vi "Configure Open Lead Detection.vi"(7 "Enable Open Lead Detection (F: Disable)":bool, 8 "error in (no error)":errorcluster, 9 "Channel List(\"\")":string, 10 "Function (5: 4-wire resistance)":i32(ring)=5 items=["4-wire Resistance"=5, "Temperature"=8], 11 "VISA resource name":refnum<visa-resource-name>) -> (0 "error out":errorcluster, 3 "VISA resource name out":refnum<visa-resource-name>)   [LabVIEW 2019, in "Keithley DMM6500 DAQ6500 Series.lvlib"]
doc: "Determines if the detection of open leads is enabled or disabled."
uses:
  Keithley DMM6500 DAQ6500 Series.lvlib
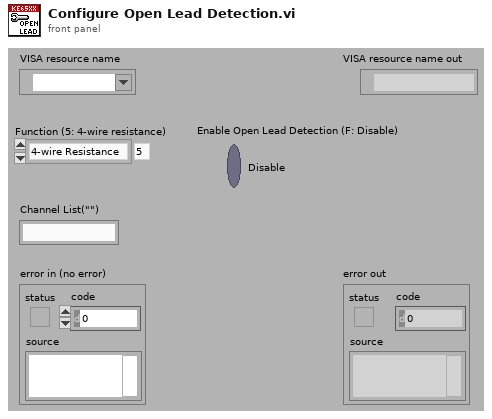
[diagram p1: front panel]
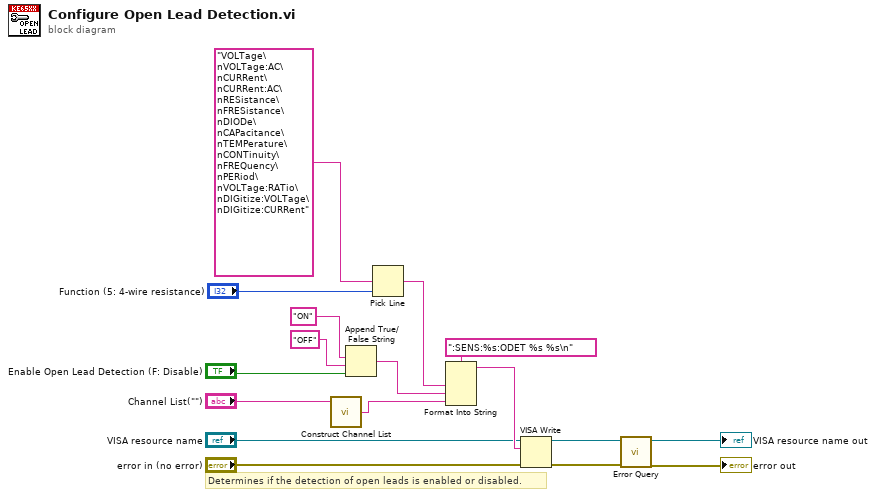
[diagram p0: block diagram]
diagram:
  # "Determines if the detection of open leads is enabled or disabled."
  n1 = call "Construct Channel List.vi"("Channel List"="Channel List(\"\")") -> ("Channel List String"=w4:string)  [unwired: 2 in]
  n2 = Append True/False String(1:"Enable Open Lead Detection (F: Disable)", 2:"OFF", 3:"ON") -> (0:w13:string)  [unwired: 1 in]
  n3 = Pick Line(multi-line string="VOLTage\nVOLTage:AC\nCURRent\nCURRent:AC\nRESistance\nFRESistance\nDIODe\nCAPacitance\nTEMPerature\nCONTinuity\nFREQuency\nPERiod\nVOLTage:RATio\nDIGitize:VOLTage\nDIGitize:CURRent", line index="Function (5: 4-wire resistance)") -> (output string=w1:string)  [unwired: 1 in]
  n4 = Format Into String(format string=":SENS:%s:ODET %s %s\n", w1, w13, w4) -> (resulting string=w12:string)  [unwired: 2 in, 1 out]
  n5 = VISA Write(VISA resource name="VISA resource name", write buffer=w12, error in (no error)="error in (no error)") -> (VISA resource name out=w9:refnum<visa-resource-name>, error out=w8:errorcluster)  [unwired: 1 out]
  n6 = call "Error Query.vi"("error in (no error)"=w8, "VISA resource name"=w9) -> ("error out"=→"error out":errorcluster, "VISA resource name out"=→"VISA resource name out":refnum<visa-resource-name>)  [unwired: 6 in, 2 out]
